vi "Construct PDU.vi"(8 "error in":errorcluster, 9 "DATA":u8[](array[numeric]), 10 "CMD_TYPE":T1(ring)=enum."CODE_CMD_POWERSTEP01") -> (0 "error out":errorcluster, 3 "SMSD data unit out":refnum<class "SMSD Data Unit.lvclass">)   [LabVIEW 2021, in "SMSD Data Unit.lvclass"]
uses:
  SMSD Data Unit.lvclass
  SMSD Data Unit.lvclass/SMSD Data Unit.ctl
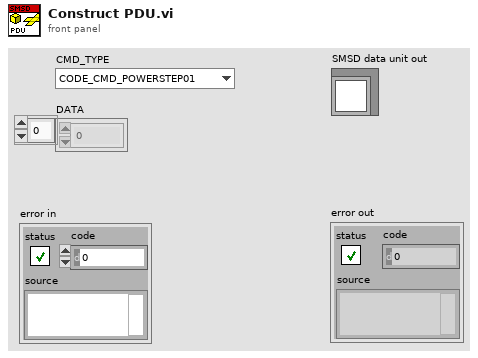
[diagram p1: front panel]
types:
  T1 = enum8{"CODE_CMD_REQUEST", "CODE_CMD_RESPONSE", "CODE_CMD_POWERSTEP01", "CODE_CMD_POWERSTEP01_W_MEM0", "CODE_CMD_POWERSTEP01_W_MEM1", "CODE_CMD_POWERSTEP01_W_MEM2", "CODE_CMD_POWERSTEP01_W_MEM3", "CODE_CMD_POWERSTEP01_R_MEM0", "CODE_CMD_POWERSTEP01_R_MEM1", "CODE_CMD_POWERSTEP01_R_MEM2", "CODE_CMD_POWERSTEP01_R_MEM3", "CODE_CMD_CONFIG_SET", "CODE_CMD_CONFIG_GET", "CODE_CMD_PASSWORD_SET", "CODE_CMD_ERROR_GET"}
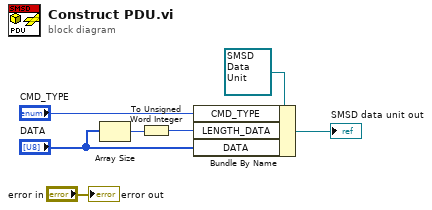
[diagram p0: block diagram]
diagram:
  n1 = Array Size(array="DATA") -> (size(s)=w5:i32)
  n2 = To Unsigned Word Integer(number=w5) -> (unsigned 16bit integer=w4:u16)
  n3 = Bundle By Name(cluster=refnum<class "SMSD Data Unit.lvclass"> refnum ("SMSD data unit"), "CMD_TYPE"="CMD_TYPE", "LENGTH_DATA"=w4, "DATA"="DATA") -> (→"SMSD data unit out":refnum<class "SMSD Data Unit.lvclass">)
  "error out" <- "error in"
